vi "Generate Post-Install.vi"() -> ()   [LabVIEW 2020]
uses:
  <vilib>/zip/NI_Unzip.lvlib
panel:
  out "error out":errorcluster
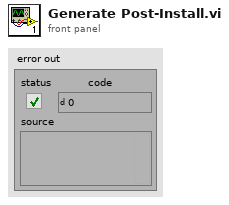
[diagram p1: front panel]
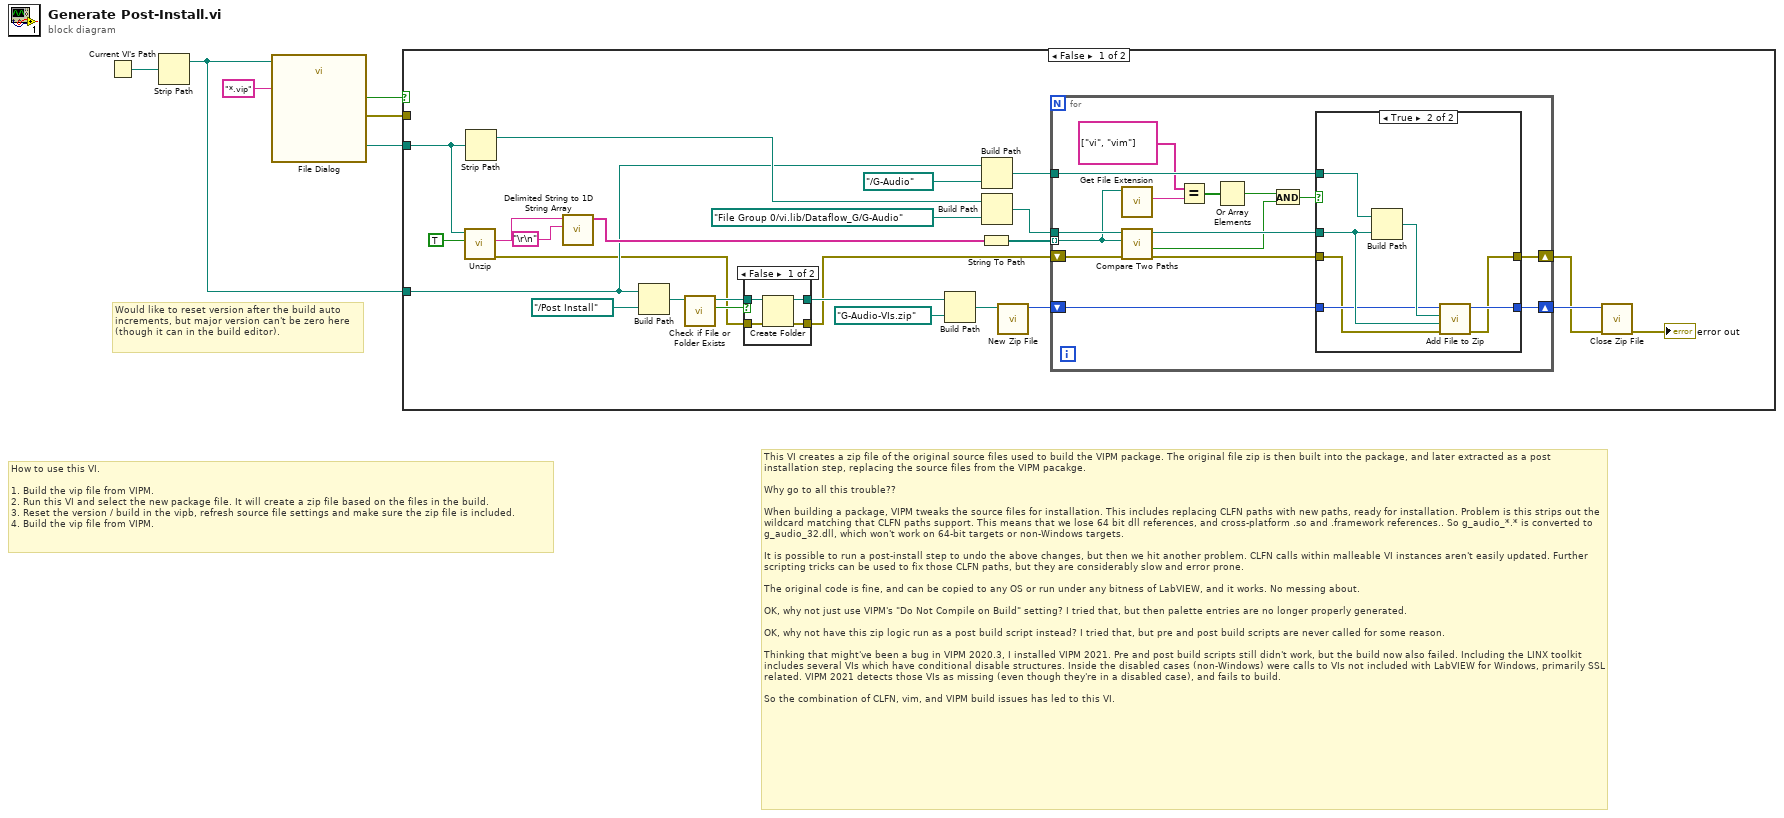
[diagram p0: block diagram]
diagram:
  # "Would like to reset version after the build auto increments, but major version can't be zero here (though it can in the build editor)."
  # "How to use this VI.\n\n1. Build the vip file from VIPM.\n2. Run this VI and select the new package file. It will create a zip file based on the files in the build.\n3. Reset the version / build in the vipb, refresh source file settings and make sure the zip file is included.\n4. Build the vip file from VIPM."
  # "This VI creates a zip file of the original source files used to build the VIPM package. The original file zip is then built into the package, and later extracted as a post installation step, replacing the source files from the VIPM pacakge.\n\nWhy go to all this trouble??\n\nWhen building a package, VIPM tweaks the source files for installation. This includes replacing CLFN paths with new paths, ready for installation. Problem is this strips out the wildcard matching that CLFN paths support. This means that we lose 64 bit dll references, and cross-platform .so and .framework references.. So g_audio_*.* is converted to g_audio_32.dll, which won't work on 64-bit targets or non-Windows targets.\n\nIt is possible to run a post-install step to undo the above changes, but then we hit another problem. CLFN calls within malleable VI instances aren't easily updated. Further scripting tricks can be used to fix those CLFN paths, but they are considerably slow and error prone.\n\nThe original code is fine, and can be copied to any OS or run under any bitness of LabVIEW, and it works. No messing about.\n\nOK, why not just use VIPM's \"Do Not Compile on Build\" setting? I tried that, but then palette entries are no longer properly generated.\n\nOK, why not have this zip logic run as a post build script instead? I tried that, but pre and post build scripts are never called for some reason.\n\nThinking that might've been a bug in VIPM 2020.3, I installed VIPM 2021. Pre and post build scripts still didn't work, but the build now also failed. Including the LINX toolkit includes several VIs which have conditional disable structures. Inside the disabled cases (non-Windows) were calls to VIs not included with LabVIEW for Windows, primarily SSL related. VIPM 2021 detects those VIs as missing (even though they're in a disabled case), and fails to build.\n\nSo the combination of CLFN, vim, and VIPM build issues has led to this VI."
  n1 = Current VI's Path() -> (path=w4:path)
  n2 = Strip Path(path=w4) -> (stripped path=w1:path)  [unwired: 1 out]
  n3 = call "File Dialog"("start path"=w1, "pattern (all files)"="*.vip") -> ("selected path"=w2:path, "cancelled"=w6:bool, "error out"=w5:errorcluster)  [unwired: 10 in, 1 out]
  n4 = case shown="False" w6 {
    tunnel: w1 -> [w13 _]
    tunnel: w5 -> [_ _]
    tunnel: w2 -> [w20 _]
    frame False {
      n5 = call <vilib>:"Unzip.vi"("Preview only?"=TRUE, "Zip file"=w20) -> ("error out"=w8:errorcluster, "Preview"=w17:string)  [unwired: 7 in, 1 out]
      n6 = Strip Path(path=w20) -> (stripped path=w19:path)  [unwired: 1 out]
      n7 = call <vilib>:"Delimited String to 1D String Array.vi"("delimiter"="\r\n", "delimited string"=w17) -> ("string array"=w15:string[])  [unwired: 9 in]
      n8 = Build Path(base path=w13, name or relative path=path "../Post Install") -> (appended path=w11:path)
      n9 = call <vilib>:"Check if File or Folder Exists.vi"("path"=w11) -> ("file or folder exists?"=w9:bool, "dup path"=w10:path)  [unwired: 8 in, 1 out]
      n10 = case shown="False" w9 {
        tunnel: [w35 w37] -> w12
        tunnel: w10 -> [w34 w37]
        tunnel: w8 -> [w33 w36]
        tunnel: [w32 w36] -> w7
        frame False {
          n11 = Create Folder(path (use dialog)=w34, error in=w33) -> (created path=w35:path, error out=w32:errorcluster)  [unwired: 1 in, 1 out]
        }
        frame True {
        }
      }
      n12 = Build Path(base path=w12, name or relative path=path "G-Audio-VIs.zip") -> (appended path=w26:path)
      n13 = String To Path(string=w15) -> (path=w21:path[])
      n14 = Build Path(base path=w13, name or relative path=path "../G-Audio") -> (appended path=w28:path)
      n15 = Build Path(base path=w19, name or relative path=path "File Group 0/vi.lib/Dataflow_G/G-Audio") -> (appended path=w30:path)
      n16 = call <vilib>:"New Zip File.vi"("target"=w26) -> ("zip file out"=w25:i64)  [unwired: 4 in, 2 out]
      n17 = for {
        tunnel: w30 -> [w39]
        tunnel: w21 -> [w38] mode=indexing
        tunnel: w28 -> [w46]
        shift-right: [w49] -> w23
        shift-left: w7 -> [w51]
        shift-right: [w47] -> w24
        shift-left: w25 -> [w48]
        n18 = call <vilib>:"Get File Extension.vi"("file"=w38) -> ("lowercase file extension"=w45:string)  [unwired: 6 in, 4 out]
        n19 = call <vilib>:"Compare Two Paths.vi"("error in (no error)"=w51, "Path 2"=w38, "Path 1"=w39) -> ("error out"=w50:errorcluster, "Path 2 Relative to Path 1?"=w43:bool, "Relative Path from 1 to 2"=w52:path)  [unwired: 5 in, 1 out]
        n20 = Equal?(x=string[] ["vi", "vim"], y=w45) -> (x = y?=w42:bool[])
        n21 = Or Array Elements(Boolean array=w42) -> (logical OR=w41:bool)
        n22 = And(x=w41, y=w43) -> (x .and. y?=w40:bool)
        n23 = case shown="True" w40 {
          tunnel: w52 -> [_ w59]
          tunnel: w46 -> [_ w61]
          tunnel: w50 -> [w54 w56]
          tunnel: [w54 w55] -> w49
          tunnel: w48 -> [w53 w58]
          tunnel: [w53 w57] -> w47
          frame False {
          }
          frame True {
            n24 = Build Path(base path=w61, name or relative path=w59) -> (appended path=w60:path)
            n25 = call <vilib>:"Add File to Zip.vi"("error in (no error)"=w56, "destination path in zip"=w59, "source file path"=w60, "zip file in"=w58) -> ("error out"=w55:errorcluster, "zip file out"=w57:i64)  [unwired: 6 in]
          }
        }
      }
      n26 = call <vilib>:"Close Zip File.vi"("error in (no error)"=w23, "zip file in"=w24) -> ("error out"=→"error out":errorcluster)  [unwired: 5 in]
    }
    frame True {
    }
  }
